vi "Analyze Enum.vi"(8 "error in (no error)":errorcluster, 11 "Enum Variant":variant) -> (0 "error dub":errorcluster, 1 "Success?":bool, 2 "Enum Alias":string, 3 "Enum Index":u32)   [LabVIEW 2020, in "Data.lvlib" / "Enum.lvclass"]
doc: "Extract 'Enum Index' and 'Enum Alias' from 'Enum Variant'. If 'Enum Variant' does not contain a valid enum 'Success?' will return FALSE."
uses:
  Enum.lvclass
  <vilib>/Utility/Data Type/NI_Data Type.lvlib
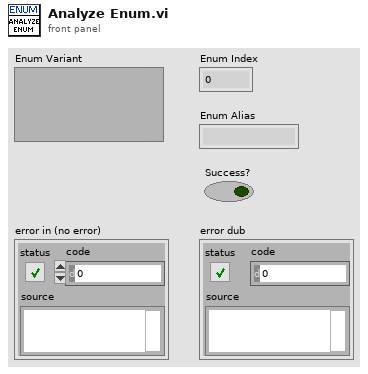
[diagram p1: front panel]
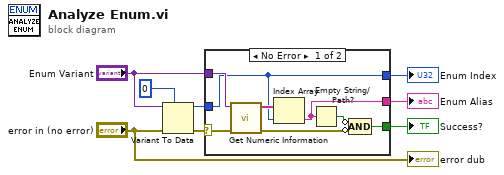
[diagram p0: block diagram]
diagram:
  n1 = Variant To Data(error in="error in (no error)", type=u32 0 ("Enum Index"), Variant="Enum Variant") -> (data=w4:u32, error out=w3:errorcluster)
  n2 = case shown="No Error" w3 {
    selector: w3 -> [w14 _]
    tunnel: w4 -> [w10 _]
    tunnel: "Enum Variant" -> [w16 _]
    tunnel: [w13 _] -> w6
    tunnel: [w10 _] -> w7
    tunnel: [w9 _] -> w8
    frame No Error {
      n3 = call <vilib>:"Get Numeric Information.vi"("error in (no error)"=w14, "variant"=w16) -> ("error out"=w11:errorcluster, "enum names"=w15:string[])  [unwired: 6 in, 2 out]
      n4 = Index Array(array=w15, index=w10) -> (element=w9:string)
      n5 = Empty String/Path?(string/path=w9) -> (empty?=w12:bool)
      n6 = Compound Arithmetic op=AND(invert w12, invert w11) -> (w13:bool)
    }
    frame Error {
    }
  }
  "Enum Alias" <- w8
  "Enum Index" <- w7
  "Success?" <- w6
  "error dub" <- "error in (no error)"
